vi "DSF.Shared.Configuration.Framework.Get Configuration Cluster.vi"(11 "Framework Configuration in":refnum<class "DSF.Shared.Configuration.Framework.lvclass">) -> (2 "Framework Configuration":T1, 3 "Framework Configuration out":refnum<class "DSF.Shared.Configuration.Framework.lvclass">)   [LabVIEW 2017, in "DSF.Shared.lvlib" / "DSF.Shared.Configuration.Framework.lvclass"]
uses:
  DSF.Shared.Configuration.Framework.lvclass
  Typedefs/DSF.Shared.Refactor.Typedefs.Framework Configuration.Aggregate.ctl
  Typedefs/DSF.Shared.Refactor.Typedefs.Plugin Configuration.Aggregate.ctl
  Typedefs/DSF.Shared.Typedefs.Cycle Timing Factors.ctl
  Typedefs/DSF.Shared.Refactor.Typedefs.Transfer Group Configuration.Aggregate.ctl
  Typedefs/DSF.Shared.Typedefs.Direction.ctl
  Typedefs/DSF.Shared.Refactor.Typedefs.Transfer Configuration.ctl
  Typedefs/DSF.Shared.Typedefs.Byte Order.ctl
  Typedefs/DSF.Shared.Refactor.Typedefs.Channel Array Configuration.ctl
  Typedefs/DSF.Shared.Typedefs.Data Type.ctl
  DSF.Shared.Configuration.Framework.lvclass/DSF.Shared.Configuration.Framework.ctl
  DSF.Shared.lvlib
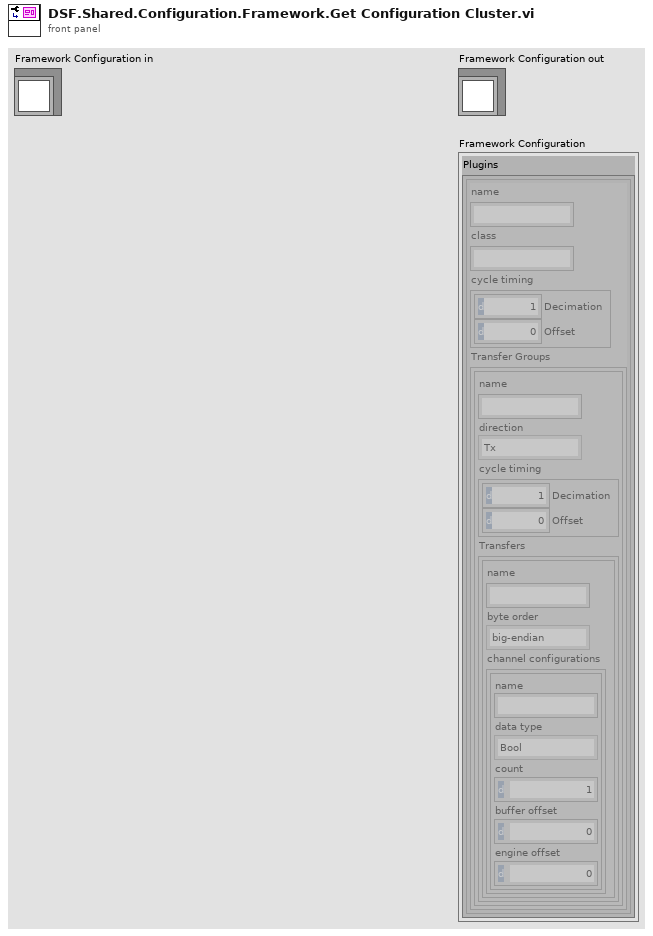
[diagram p1: front panel]
types:
  T1 = typedef "DSF.Shared.lvlib/DSF.Shared.Refactor.Typedefs.Framework Configuration.Aggregate.ctl" = cluster{"Plugins":T2[]}
  T2 = typedef "DSF.Shared.lvlib/DSF.Shared.Refactor.Typedefs.Plugin Configuration.Aggregate.ctl" = cluster{"name":string, "class":string, "cycle timing":T3, "Transfer Groups":T4[]}
  T3 = typedef "DSF.Shared.lvlib/DSF.Shared.Typedefs.Cycle Timing Factors.ctl" = cluster{"Decimation":u64, "Offset":u64}
  T4 = typedef "DSF.Shared.lvlib/DSF.Shared.Refactor.Typedefs.Transfer Group Configuration.Aggregate.ctl" = cluster{"name":string, "direction":T5, "cycle timing":T3, "Transfers":T6[]}
  T5 = typedef "DSF.Shared.lvlib/DSF.Shared.Typedefs.Direction.ctl" = enum8{"Tx", "Rx"}
  T6 = typedef "DSF.Shared.lvlib/DSF.Shared.Refactor.Typedefs.Transfer Configuration.ctl" = cluster{"name":string, "byte order":T7, "channel configurations":T8[]}
  T7 = typedef "DSF.Shared.lvlib/DSF.Shared.Typedefs.Byte Order.ctl" = enum8{"big-endian", "little-endian"}
  T8 = typedef "DSF.Shared.lvlib/DSF.Shared.Refactor.Typedefs.Channel Array Configuration.ctl" = cluster{"name":string, "data type":T9, "count":u64, "buffer offset":u64, "engine offset":u64}
  T9 = typedef "DSF.Shared.lvlib/DSF.Shared.Typedefs.Data Type.ctl" = enum8{"Bool", "SGL", "DBL", "I8", "I16", "I32", "I64", "U8", "U16", "U32", "U64"}
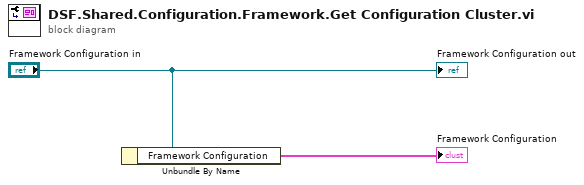
[diagram p0: block diagram]
diagram:
  n1 = Unbundle By Name("Framework Configuration in") -> ("Framework Configuration"=→"Framework Configuration":T1)
  "Framework Configuration out" <- "Framework Configuration in"
